vi "lv-build.vi"() -> (0 "error out":errorcluster)   [LabVIEW 2014, in "lv-build-library.lvlib"]
uses:
  lv-build-library.lvlib
  <vilib>/Utility/error.llb/DialogType.ctl
  <vilib>/AppBuilder/AB_API_Simple/Build (path).vi
  <vilib>/Wiresmith Technology/LabVIEW CLI/CLI Class/CLI.lvclass
  <vilib>/AppBuilder/AB_API_Simple/NI_App_Builder_API.lvlib
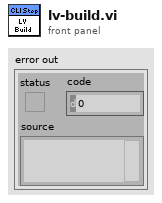
[diagram p1: front panel]
types:
  T1 = typedef "DialogType.ctl" = u16
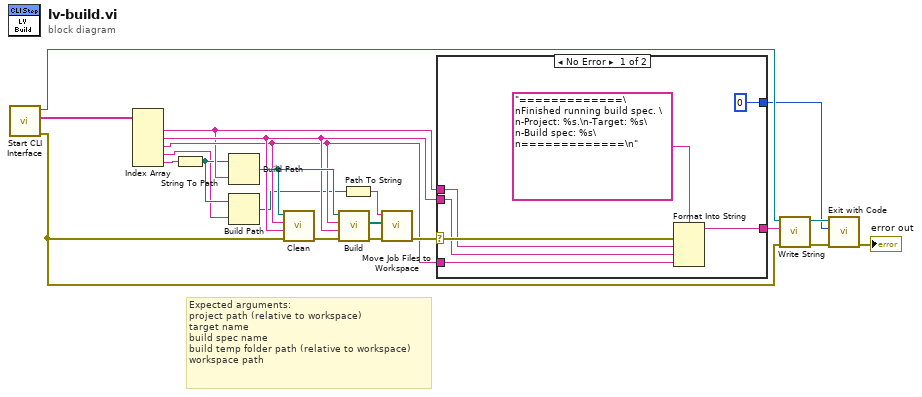
[diagram p0: block diagram]
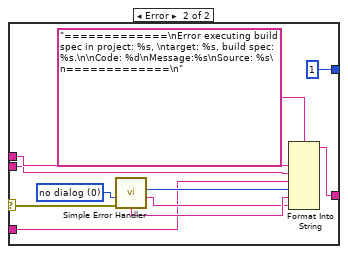
[diagram p2: hidden frame]
diagram:
  # "Expected arguments:\nproject path (relative to workspace)\ntarget name\nbuild spec name\nbuild temp folder path (relative to workspace)\nworkspace path"
  n1 = call <vilib>:"Start CLI Interface.vi"() -> ("error out"=w7:errorcluster, "Custom Parameters"=w21:string[], "CLI out"=w19:refnum<class "CLI.lvclass">)  [unwired: 9 in]
  n2 = Index Array(array=w21) -> (element #1=w6:string, element #2=w9:string, element #3=w8:string, element #4=w3:string, element #5=w5:string)  [unwired: 5 in]
  n3 = String To Path(string=w5) -> (path=w4:path)
  n4 = Build Path(base path=w4, name or relative path=w6) -> (appended path=w10:path)
  n5 = Build Path(base path=w4, name or relative path=w3) -> (appended path=w1:path)
  n6 = call <vilib>:"Clean.vi"("error in (no error)"=w7, "Name of target (My Computer)"=w9, "Name of build specification (if empty: clean all)"=w8, "Path to project"=w10) -> ("error out"=w13:errorcluster)  [unwired: 7 in]
  n7 = call-poly <vilib>:"Build.vi"("error in (no error)"=w13, "Name of target (My Computer)"=w9, "Name of build specification (if empty: build all)"=w8, "Path to project"=w10) -> ("error out"=w12:errorcluster, "Generated files"=w11:path[])  [unwired: 6 in]
  n8 = Path To String(path=w1) -> (string=w2:string)
  n9 = call "Move Job Files to Workspace.vi"("error in (no error)"=w12, "Generated Files"=w11, "Workspace Path"=w2) -> ("error out"=w15:errorcluster)  [unwired: 8 in]
  n10 = case shown="No Error" w15 {
    selector: w15 -> [w27 w38]
    tunnel: w6 -> [w26 w31]
    tunnel: w9 -> [w25 w30]
    tunnel: [w24 w39] -> w20
    tunnel: [0 ("Exit Code (0)") 1 ("Exit Code (0)")] -> w16
    tunnel: w8 -> [w22 w29]
    frame No Error {
      n11 = Format Into String(format string="=============\nFinished running build spec. \n-Project: %s.\n-Target: %s\n-Build spec: %s\n=============\n", error in=w27, w26, w25, w22) -> (resulting string=w24:string)  [unwired: 1 in, 1 out]
    }
    frame Error {
      w37 = T1 0 items=["no dialog", "OK message", "continue or stop message", "OK message + warnings", "continue/stop + warnings"] ("type of dialog (OK msg:1)")
      n12 = call <vilib>:"Simple Error Handler.vi"("type of dialog (OK msg:1)"=w37, "error in (no error)"=w38) -> ("code out"=w32:i32, "source out"=w33:string, "message"=w34:string)  [unwired: 3 in, 2 out]
      n13 = Format Into String(format string="=============\nError executing build spec in project: %s, \ntarget: %s, build spec: %s.\n\nCode: %d\nMessage:%s\nSource: %s\n=============\n", w31, w30, w29, w32, w34, w33) -> (resulting string=w39:string)  [unwired: 2 in, 1 out]
    }
  }
  n14 = call <vilib>:"Write String.vi"("error in (no error)"=w7, "Text to Write"=w20, "CLI in"=w19) -> ("error out"=w18:errorcluster, "CLI out"=w17:refnum<class "CLI.lvclass">)  [unwired: 7 in]
  n15 = call <vilib>:"Exit with Code.vi"("error in (no error)"=w18, "Exit Code (0)"=w16, "CLI in"=w17) -> ("error out"=→"error out":errorcluster)  [unwired: 8 in]
